vi "Is Chassis Active.vi"(8 "error in":errorcluster, 11 "SL_SC in":refnum<class "SL_SC.lvclass">) -> (0 "error out":errorcluster, 2 "Chassis Active":bool, 3 "SL_SC out":refnum<class "SL_SC.lvclass">)   [LabVIEW 2019]
uses:
  <vilib>/SLSC/SLSC.lvlib
  <resource>/objmgr/slsc.rc
  <vilib>/SLSC/Initialize Session without Resources.vi
  <vilib>/SLSC/Close Session.vi
  Library/SL_SC.lvclass
  C:/Users/Public/Documents/Development/builds/Instruments/DIG_IO.lvlibp/Library/DIG_IO.lvclass
  C:/Users/Public/Documents/Development/builds/Instruments/Instruments.lvlibp/Library/Instruments.lvclass
  C:/Users/Public/Documents/Development/builds/Tools/Config.lvlibp/Config.lvclass
  C:/Users/Public/Documents/Development/builds/Engine/Engine.lvlibp/Project/Engine.lvclass
  C:/Users/Public/Documents/Development/builds/Engine/State Actor.lvlibp/Library/State Actor.lvclass
  C:/Users/Public/Documents/Development/builds/Engine/Panel Manager.lvlibp/Panel Actor/Panel Actor.lvclass
  C:/Users/Public/Documents/Development/builds/Engine/Monitored Actor.lvlibp/Monitored Actor/Monitored Actor/Monitored Actor.lvclass
  C:/Users/Public/Documents/Development/builds/Engine/Actor Framework.lvlibp/1abvi3w/vi.lib/ActorFramework/Actor/Actor.lvclass
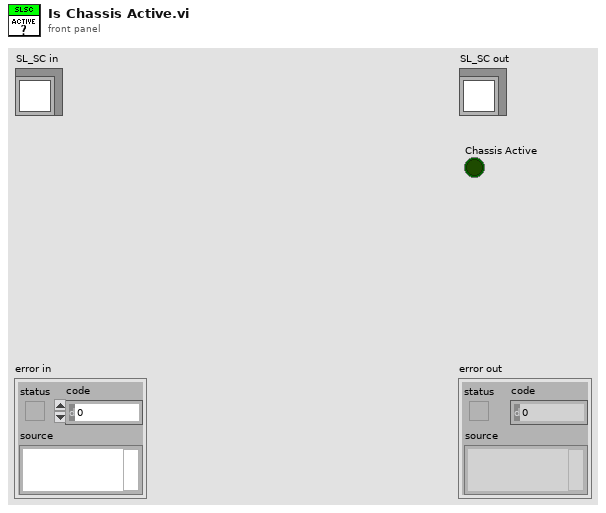
[diagram p1: front panel]
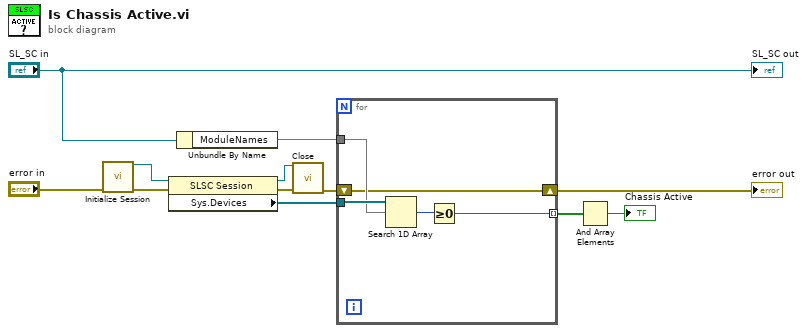
[diagram p0: block diagram]
diagram:
  n1 = call-poly <vilib>:"Initialize Session.vi"("error in (no error)"="error in") -> ("session out"=w10:refnum<k21>, "error out"=w11:errorcluster)  [unwired: 13 in]
  n2 = property class="SLSC Session"(reference=w10, error in=w11) -> (reference out=w4:refnum<k21>, error out=w5:errorcluster, "Sys.Devices"=w8:refnum<k21>[])
  n3 = Unbundle By Name("SL_SC in") -> ("ModuleNames"=w7)
  n4 = call-poly <vilib>:"Close.vi"("session in"=w4, "error in (no error)"=w5) -> ("error out"=w3:errorcluster)  [unwired: 13 in]
  n5 = for {
    tunnel: w8 -> [w17]
    tunnel: w7 -> [w16]
    tunnel: [w14] -> w6 mode=indexing
    shift-right: [w13] -> w2
    shift-left: w3 -> [w13]
    n6 = Search 1D Array(1D array=w17, element=w16) -> (index of element=w15:i32)  [unwired: 1 in]
    n7 = Greater Or Equal To 0?(x=w15) -> (x >= 0?=w14:bool)
  }
  "error out" <- w2
  n8 = And Array Elements(Boolean array=w6) -> (logical AND=→"Chassis Active":bool)
  "SL_SC out" <- "SL_SC in"
